vi "TPP-printer-v3.1.vi"() -> ()   [LabVIEW 2015]
uses:
  <vilib>/DAQmx/write.llb/DAQmx Write (Digital Bool 1Line 1Point).vi
  <vilib>/Utility/file.llb/Read Delimited Spreadsheet (I64).vi
  <vilib>/DAQmx/create/channels.llb/DAQmx Create Channel (DO-Digital Output).vi
  <vilib>/DAQmx/miscellaneous.llb/DAQmx Fill In Error Info.vi
  <vilib>/Platform/NI_3dgraph.lvlib
  Kinesis/Thorlabs.MotionControl.Controls.dll
panel:
  out "层时间":timestamp
  out "行时间":timestamp
  out "点时间":timestamp
  in  "f_objecitve(mm)":dbl=1.8
  in  "f_tubelens(mm)":dbl=200.0
  in  "f_scanlens(mm)":dbl=50.0
  out "%":dbl=1.1971958040155672 format="%#.2g"
  in  "读取点阵文件":path=path "C:/Users/Hongq/Desktop/grating.txt"
  in  "停止":bool
  out "每层耗时/s":dbl format="%#.2g"
  out "每行耗时/s":dbl=0.4888782501220703 format="%#.2g"
  out "每点耗时/ms":dbl=4.009246826171875 format="%#.0f"
  out "当前完成量：":u8(slide)=1 scale=0.0..100.0
  out "耗时/min":dbl=0.11883490880330404 format="%#.2g"
  out "模型XYZG坐标表":dbl[][](array[numeric])
  in  "模型高/um":dbl=1.0
  in  "总体预览":refnum<k7>(container)
  in  "刷新预览":bool
  in  "Z轴驱动序列号":string="27000001"
  in  "KCubeDCServoControl":refnum<k24>(container)
  in  "XY速度(um/s)":dbl
  out "XYZG当前值/um":dbl[](array[numeric])=[-0.4166666666666667, -0.1875, 0.0, 7.132113933563232, 7.091063499450684, 0.0] format="%#.2g"
  in  "比例因子(V/°)":dbl=0.5
  in  "AO通道：X前Y后":tag="Dev1/ao0:1"
  out "当前扫描速度(um/s)":dbl
  in  "DO通道：shutter控制":tag="Dev1/port1/line0" caption="线"
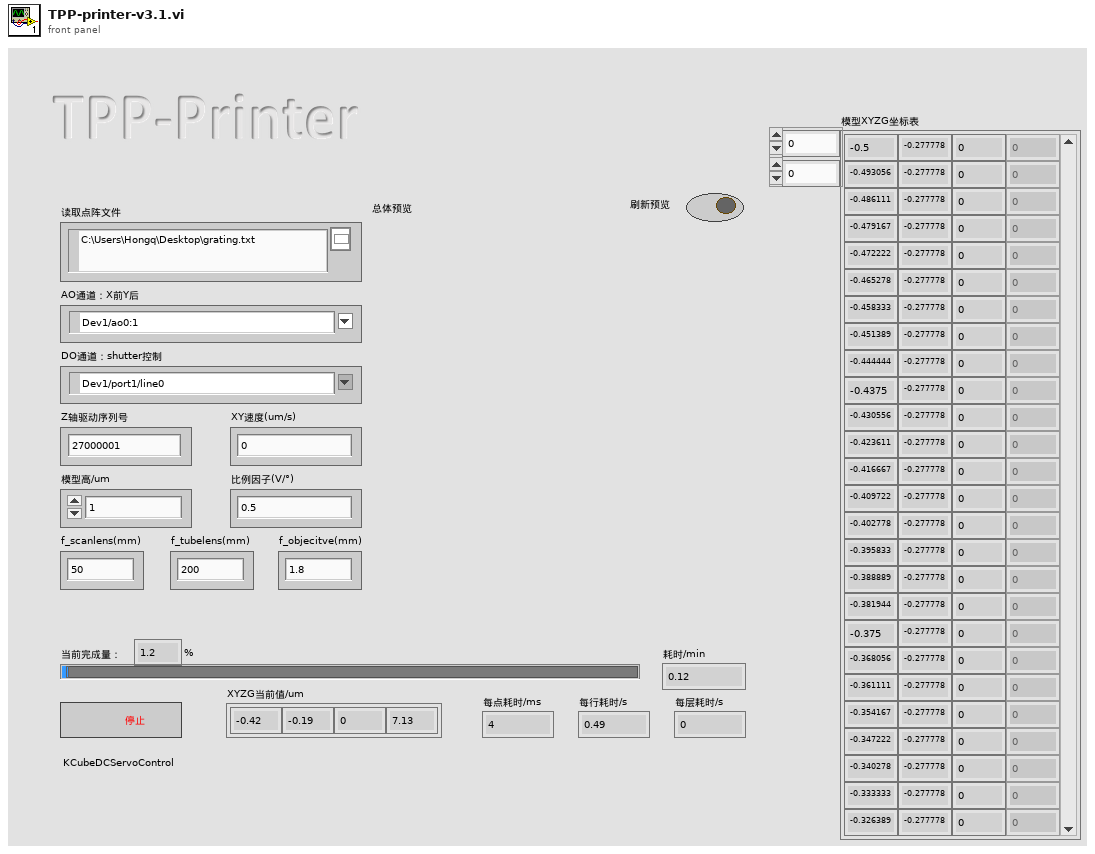
[diagram p1: front panel]
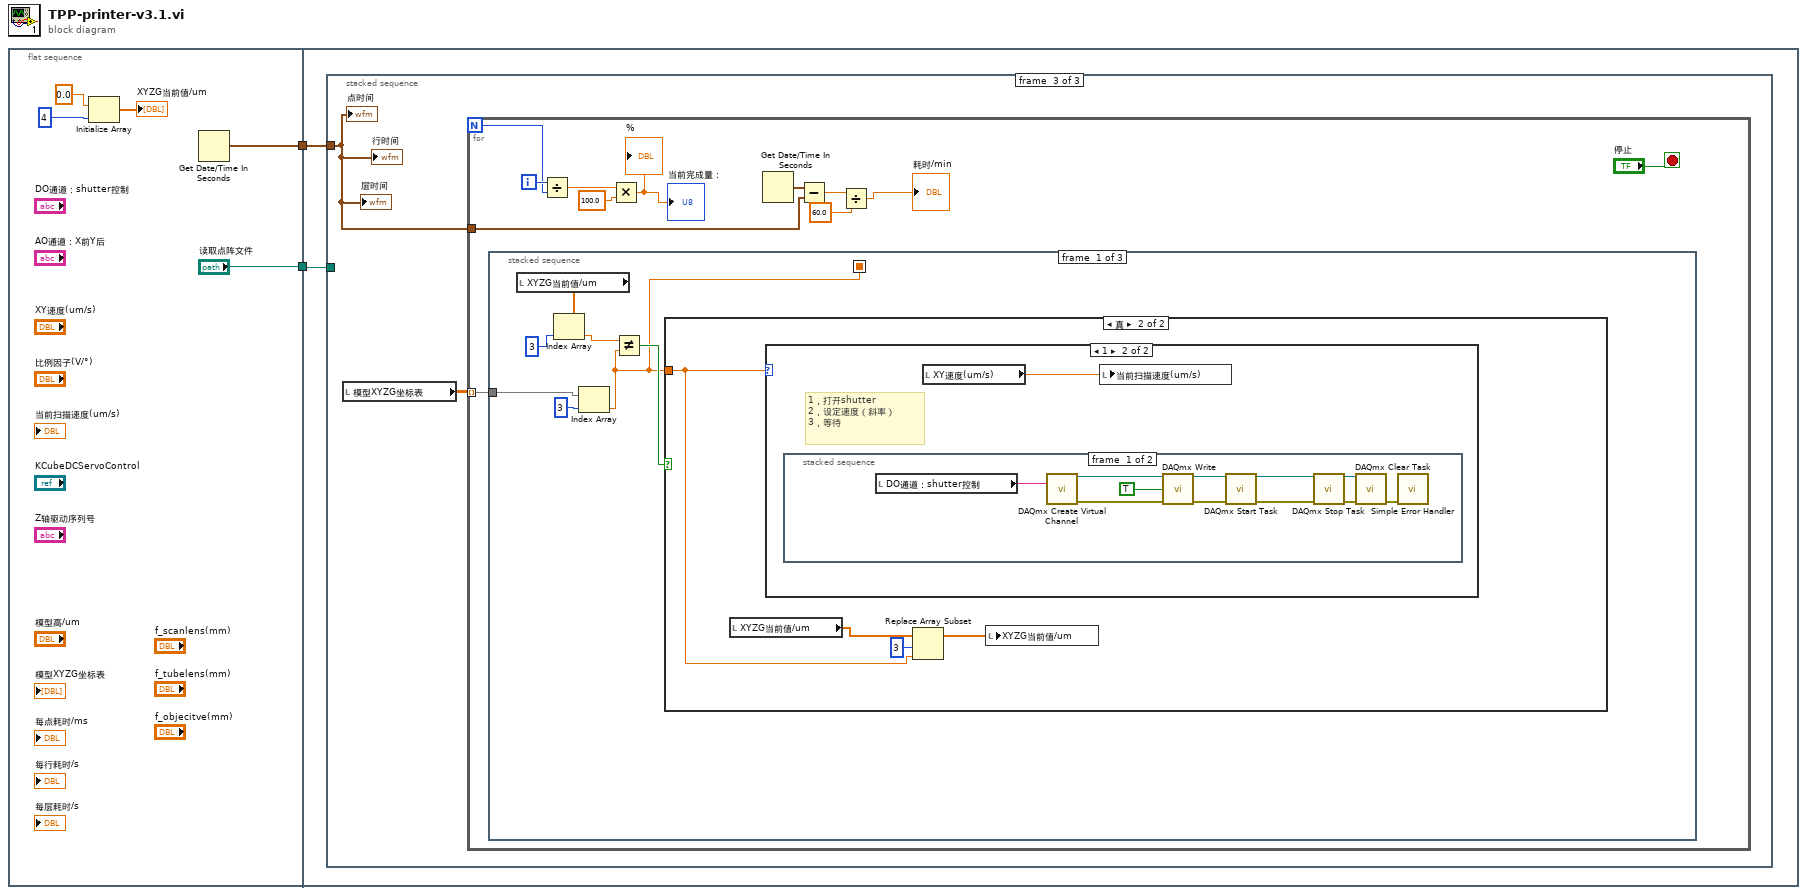
[diagram p0: block diagram]
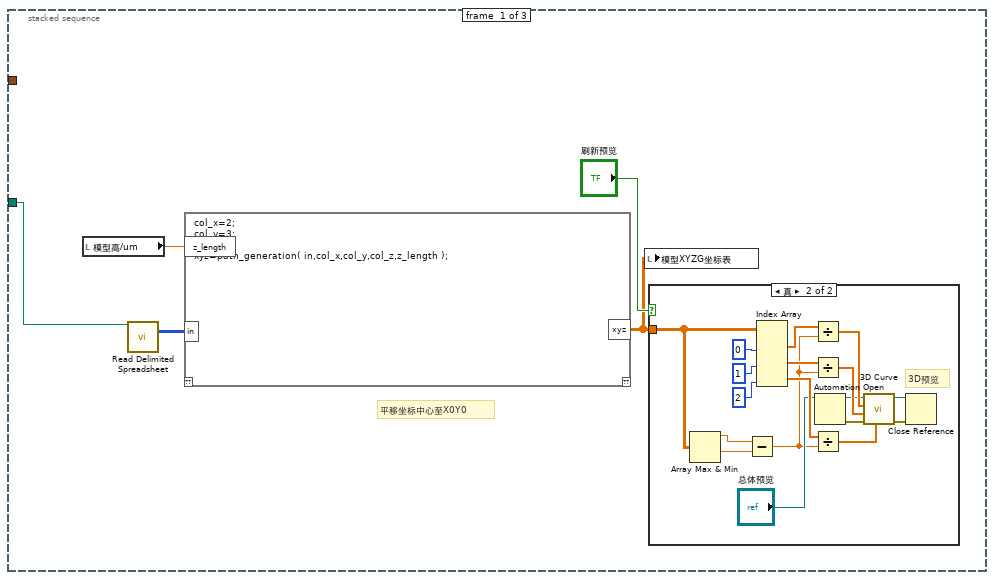
[diagram p2: hidden frame]
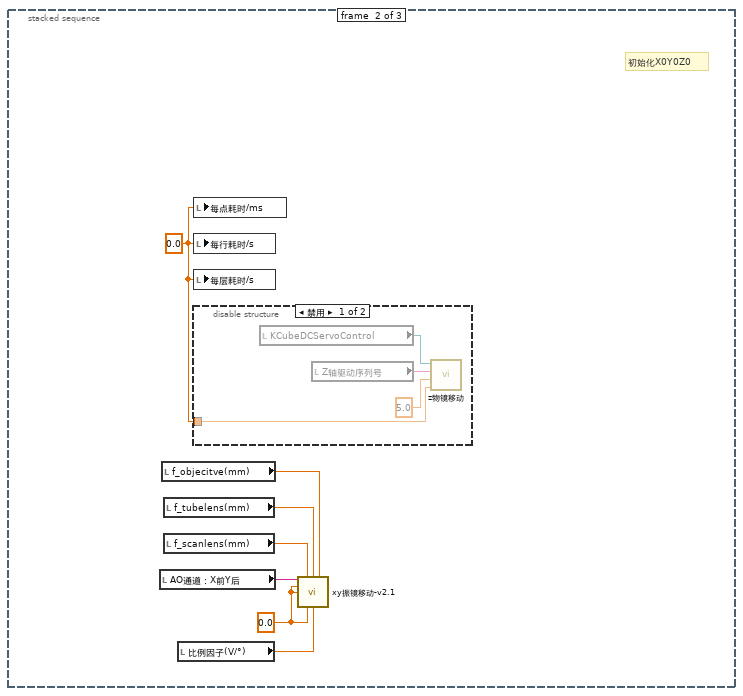
[diagram p4: hidden frame]
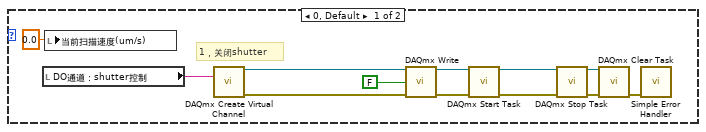
[diagram p7: hidden frame]
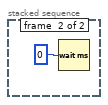
[diagram p8: hidden frame]
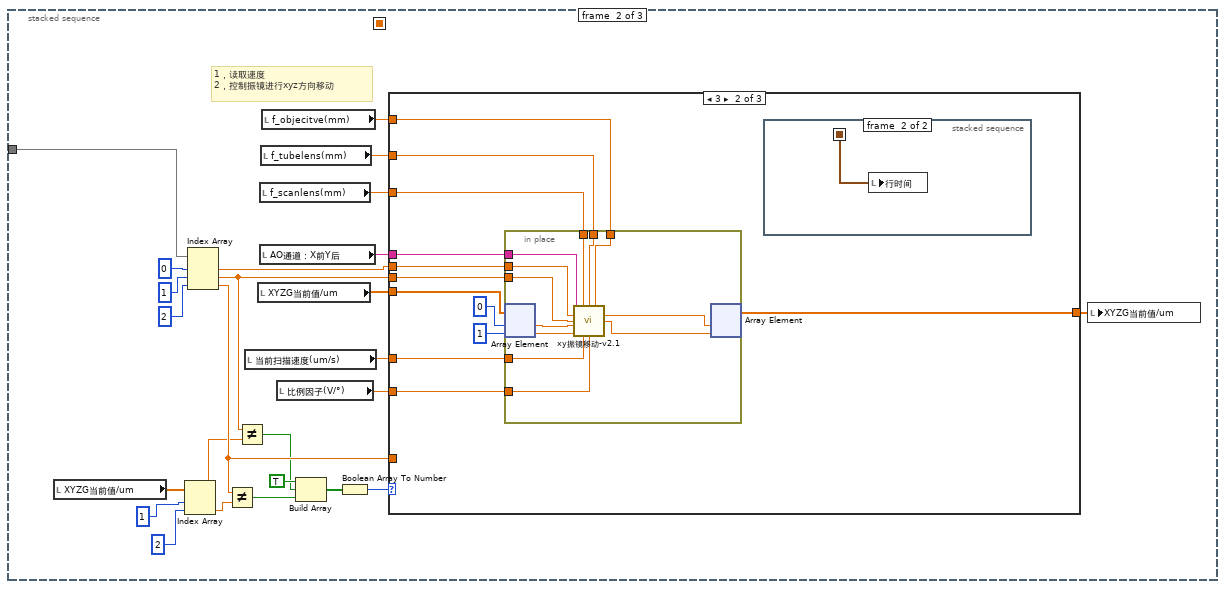
[diagram p9: hidden frame]
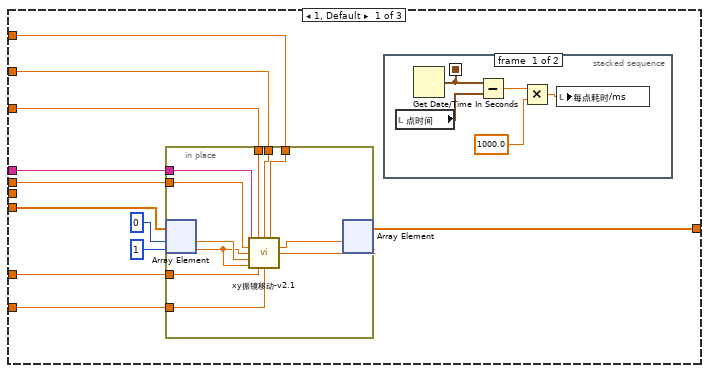
[diagram p10: hidden frame]
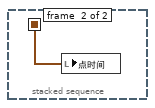
[diagram p11: hidden frame]
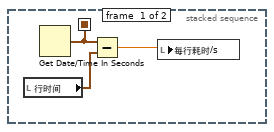
[diagram p12: hidden frame]
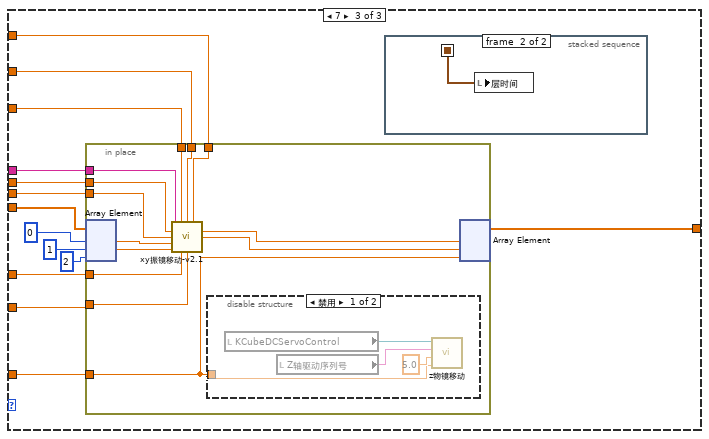
[diagram p13: hidden frame]
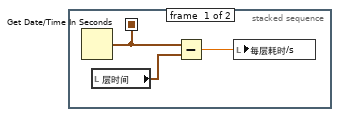
[diagram p14: hidden frame]
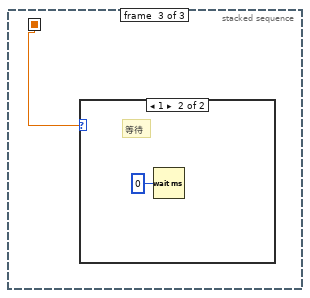
[diagram p16: hidden frame]
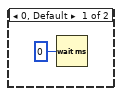
[diagram p17: hidden frame]
diagram:
  n1 = flat-sequence {
    tunnel: [w4] -> w2
    tunnel: ["读取点阵文件"] -> w1
    tunnel: w2 -> [w9]
    tunnel: w1 -> [w8]
    frame #0 {
      n2 = Initialize Array(0.0 ("元素"), 4 ("维数大小")) -> (→"XYZG当前值/um":dbl[])
      n3 = Get Date/Time In Seconds() -> (seconds since 1Jan1904=w4:timestamp)
    }
    frame #1 {
      n4 = stacked-sequence {
        tunnel: w9 -> [_ _ w44]
        tunnel: w8 -> [w13 _ _]
        frame #0 {
          # "平移坐标中心至X0Y0"
          n5 = local read "模型高/um"() -> (w11:dbl)
          n6 = call-poly <vilib>:"Read Delimited Spreadsheet.vi"("file path (dialog if empty)"=w13) -> ("all rows"=w12:i64[][])  [unwired: 9 in, 5 out]
          n7 = script code="col_x=2;\ncol_y=3;\ncol_z=4;\nxyz=path_generation( in,col_x,col_y,col_z,z_length );"("in"=w12, "z_length"=w11) -> ("xyz"=w10:dbl[][])  [unwired: 1 in, 1 out]
          n8 = local write "模型XYZG坐标表"(w10) -> ()
          n9 = case shown="真" "刷新预览" {
            tunnel: w10 -> [_ w18]
            frame False {
            }
            frame True {
              # "3D预览"
              n10 = Array Max & Min(array=w18) -> (max value=w16:dbl, min value=w17:dbl)  [unwired: 2 out]
              n11 = Subtract(x=w16, y=w17) -> (x-y=w15:dbl)
              n12 = Index Array(array=w18, index (col) #1=0 ("禁用的索引 (列)"), index (col) #2=1 ("索引 (列)"), index (col) #3=2 ("索引 (列)")) -> (element #1=w29:dbl[], element #2=w28:dbl[], element #3=w27:dbl[])  [unwired: 3 in]
              n13 = Divide(x=w29, y=w15) -> (x/y=w24:dbl[])
              n14 = Divide(x=w28, y=w15) -> (x/y=w25:dbl[])
              n15 = Divide(x=w27, y=w15) -> (x/y=w26:dbl[])
              n16 = Automation Open(Automation Refnum="总体预览") -> (Automation Refnum=w22:refnum<k7>, error out=w19:errorcluster)  [unwired: 3 in]
              n17 = call <vilib>:"3D Curve.vi"("z vector"=w26, "error in (no error)"=w19, "y vector"=w25, "x vector"=w24, "3D graph"=w22) -> ("error out"=w21:errorcluster, "3D graph out"=w20:refnum<k7>)  [unwired: 5 in]
              n18 = Close Reference(reference=w20, error in (no error)=w21) -> ()  [unwired: 1 out]
            }
          }
        }
        frame #1 {
          w34 = 0.0 ("每点耗时/ms")
          w33 = 0.0 ("速度(°/s)")
          # "初始化X0Y0Z0"
          n19 = local read "AO通道：X前Y后"() -> (w39:tag)
          n20 = local read "f_objecitve(mm)"() -> (w35:dbl)
          n21 = local read "f_tubelens(mm)"() -> (w36:dbl)
          n22 = local read "f_scanlens(mm)"() -> (w37:dbl)
          n23 = local read "比例因子(V/°)"() -> (w38:dbl)
          n24 = local write "每点耗时/ms"(w34) -> ()
          n25 = local write "每行耗时/s"(w34) -> ()
          n26 = local write "每层耗时/s"(w34) -> ()
          n27 = disable-structure shown="禁用" {
            disable-tunnel: w34 -> [w40 _]
            frame Disabled {
              n28 = local read "KCubeDCServoControl"() -> (w43:refnum<k24>)
              n29 = local read "Z轴驱动序列号"() -> (w42:string)
              n30 = call "z物镜移动.vi"("position"=w40, "maxVelocity"=5.0, "SerialNumber"=w42, "KCubeDCServoControl"=w43) -> ()  [unwired: 5 in, 3 out]
            }
            frame Enabled {
            }
          }
          n31 = call "xy振镜移动-v2.1.vi"("AO通道：X前Y后"=w39, "f_scanlens(mm)"=w37, "f_tubelens(mm)"=w36, "f_objecitve(mm)"=w35, "x终止位(um)"=w33, "y终止位(um)"=w33, "速度(um/s)"=w33, "比例因子(V/°)"=w38) -> ()  [unwired: 6 in, 2 out]
        }
        frame #2 {
          n32 = local read "模型XYZG坐标表"() -> (w45:dbl[][])
          n33 = for {
            N -> [w55]
            tunnel: w45 -> [w57] mode=indexing
            tunnel: w44 -> [w51]
            i -> [w56]
            stop <- "停止" stop-if-true
            n34 = stacked-sequence {
              seq-local: [w58 _ _] -> [_ _ w210]
              tunnel: w57 -> [w63 w117 _]
              frame #0 {
                n35 = local read "XYZG当前值/um"() -> (w61:dbl[])
                n36 = Index Array(array=w61, index=3 ("索引")) -> (element=w59:dbl)
                n37 = Index Array(array=w63, index=3 ("禁用的索引 (列)")) -> (element=w58:dbl)
                n38 = Not Equal?(x=w59, y=w58) -> (x != y?=w62:bool)
                n39 = case shown="真" w62 {
                  tunnel: w58 -> [_ w66]
                  frame False {
                  }
                  frame True {
                    n40 = local read "XYZG当前值/um"() -> (w68:dbl[])
                    n41 = case shown="1" w66 {
                      frame 0, Default {
                        # "1，关闭shutter"
                        n42 = local read "DO通道：shutter控制"() -> (w72:tag)
                        n43 = local write "当前扫描速度(um/s)"(0.0 ("扫描速度(°/s)")) -> ()
                        n44 = call-poly <vilib>:"DAQmx Create Virtual Channel.vi"("lines"=w72) -> ("task out"=w80:refnum<k21>, "error out"=w79:errorcluster)  [unwired: 13 in]
                        n45 = call-poly <vilib>:"DAQmx Write.vi"("task/channels in"=w80, "data"=FALSE, "error in"=w79) -> ("task out"=w77:refnum<k21>, "error out"=w76:errorcluster)  [unwired: 10 in, 1 out]
                        n46 = call <vilib>:"DAQmx Start Task.vi"("task/channels in"=w77, "error in"=w76) -> ("task out"=w70:refnum<k21>, "error out"=w69:errorcluster)  [unwired: 12 in]
                        n47 = call <vilib>:"DAQmx Stop Task.vi"("task/channels in"=w70, "error in"=w69) -> ("task out"=w75:refnum<k21>, "error out"=w74:errorcluster)  [unwired: 12 in]
                        n48 = call <vilib>:"DAQmx Clear Task.vi"("task in"=w75, "error in"=w74) -> ("error out"=w73:errorcluster)  [unwired: 13 in]
                        n49 = call <vilib>:"Simple Error Handler.vi"("error in (no error)"=w73) -> ()  [unwired: 4 in, 5 out]
                      }
                      frame 1 {
                        # "1，打开shutter\n2，设定速度（斜率）\n3，等待"
                        n50 = stacked-sequence {
                          frame #0 {
                            n51 = local read "DO通道：shutter控制"() -> (w84:tag)
                            n52 = call-poly <vilib>:"DAQmx Create Virtual Channel.vi"("lines"=w84) -> ("task out"=w92:refnum<k21>, "error out"=w91:errorcluster)  [unwired: 13 in]
                            n53 = call-poly <vilib>:"DAQmx Write.vi"("task/channels in"=w92, "data"=TRUE, "error in"=w91) -> ("task out"=w89:refnum<k21>, "error out"=w88:errorcluster)  [unwired: 10 in, 1 out]
                            n54 = call <vilib>:"DAQmx Start Task.vi"("task/channels in"=w89, "error in"=w88) -> ("task out"=w83:refnum<k21>, "error out"=w82:errorcluster)  [unwired: 12 in]
                            n55 = call <vilib>:"DAQmx Stop Task.vi"("task/channels in"=w83, "error in"=w82) -> ("task out"=w87:refnum<k21>, "error out"=w86:errorcluster)  [unwired: 12 in]
                            n56 = call <vilib>:"DAQmx Clear Task.vi"("task in"=w87, "error in"=w86) -> ("error out"=w85:errorcluster)  [unwired: 13 in]
                            n57 = call <vilib>:"Simple Error Handler.vi"("error in (no error)"=w85) -> ()  [unwired: 4 in, 5 out]
                          }
                          frame #1 {
                            n58 = Wait (ms)(milliseconds to wait=u32 0 ("等待时间（毫秒）")) -> ()  [unwired: 1 out]
                          }
                        }
                        n59 = local read "XY速度(um/s)"() -> (w81:dbl)
                        n60 = local write "当前扫描速度(um/s)"(w81) -> ()
                      }
                    }
                    n61 = Replace Array Subset(array=w68, new element=w66, index=3 ("索引")) -> (w65:dbl[])
                    n62 = local write "XYZG当前值/um"(w65) -> ()
                  }
                }
              }
              frame #1 {
                # "1，读取速度\n2，控制振镜进行xyz方向移动"
                n63 = local read "XYZG当前值/um"() -> (w104:dbl[])
                n64 = Index Array(array=w104, index #1=1 ("索引"), index #2=2 ("索引")) -> (element #1=w95:dbl, element #2=w97:dbl)
                n65 = Index Array(array=w117, index #1=0 ("禁用的索引 (列)"), index #2=1 ("索引"), index #3=2 ("索引")) -> (element #1=w108:dbl, element #2=w96:dbl, element #3=w103:dbl)
                n66 = Not Equal?(x=w103, y=w97) -> (x != y?=w102:bool)
                n67 = Not Equal?(x=w96, y=w95) -> (x != y?=w94:bool)
                n68 = local read "当前扫描速度(um/s)"() -> (w114:dbl)
                n69 = local read "XYZG当前值/um"() -> (w112:dbl[])
                n70 = local read "f_scanlens(mm)"() -> (w101:dbl)
                n71 = local read "AO通道：X前Y后"() -> (w116:tag)
                n72 = local read "f_tubelens(mm)"() -> (w100:dbl)
                n73 = local read "f_objecitve(mm)"() -> (w99:dbl)
                n74 = local read "比例因子(V/°)"() -> (w115:dbl)
                n75 = Build Array(TRUE ("元素"), w94, w102) -> (w110:bool[])
                n76 = Boolean Array To Number(Boolean array=w110) -> (number=w111:u32)
                n77 = case shown="3" w111 {
                  tunnel: w116 -> [w124 w153 w185]
                  tunnel: w115 -> [w123 w152 w186]
                  tunnel: w108 -> [w126 w154 w184]
                  tunnel: w112 -> [w129 w155 w183]
                  tunnel: [w119 w147 w175] -> w113
                  tunnel: w114 -> [w125 w156 w182]
                  tunnel: w96 -> [_ w151 w181]
                  tunnel: w103 -> [_ _ w176]
                  tunnel: w101 -> [w122 w150 w180]
                  tunnel: w100 -> [w121 w149 w179]
                  tunnel: w99 -> [w120 w148 w178]
                  frame 1, Default {
                    n78 = in-place {
                      in-place-border: w126 -> [w140]
                      in-place-border: w125 -> [w146]
                      in-place-border: w124 -> [w145]
                      in-place-border: w123 -> [w144]
                      in-place-border: w122 -> [w143]
                      in-place-border: w121 -> [w142]
                      in-place-border: w120 -> [w141]
                      n79 = in-place-array #1(w129, 0, 1) -> (w139:dbl, w138:dbl)
                      n80 = call "xy振镜移动-v2.1.vi"("AO通道：X前Y后"=w145, "f_scanlens(mm)"=w143, "f_tubelens(mm)"=w142, "f_objecitve(mm)"=w141, "x终止位(um)"=w140, "y终止位(um)"=w138, "x初始位(um)"=w139, "y初始位(um)"=w138, "速度(um/s)"=w146, "比例因子(V/°)"=w144) -> ("x终止位(um) 2"=w137:dbl, "y终止位(um) 2"=w136:dbl)  [unwired: 4 in]
                      n81 = in-place-array #1(w137, w136) -> (w119:dbl[])  [unwired: 2 out]
                    }
                    n82 = stacked-sequence {
                      seq-local: [w130 _] -> [_ w135]
                      frame #0 {
                        n83 = local read "点时间"() -> (w131:timestamp)
                        n84 = Get Date/Time In Seconds() -> (seconds since 1Jan1904=w130:timestamp)
                        n85 = Subtract(x=w130, y=w131) -> (x-y=w134:dbl)
                        n86 = Multiply(x=w134, y=1000.0) -> (x*y=w132:dbl)
                        n87 = local write "每点耗时/ms"(w132) -> ()
                      }
                      frame #1 {
                        n88 = local write "点时间"(w135) -> ()
                      }
                    }
                  }
                  frame 3 {
                    n89 = in-place {
                      in-place-border: w154 -> [w174]
                      in-place-border: w156 -> [w173]
                      in-place-border: w153 -> [w172]
                      in-place-border: w152 -> [w171]
                      in-place-border: w151 -> [w167]
                      in-place-border: w150 -> [w170]
                      in-place-border: w149 -> [w169]
                      in-place-border: w148 -> [w168]
                      n90 = in-place-array #2(w155, 0, 1) -> (w166:dbl, w165:dbl)
                      n91 = call "xy振镜移动-v2.1.vi"("AO通道：X前Y后"=w172, "f_scanlens(mm)"=w170, "f_tubelens(mm)"=w169, "f_objecitve(mm)"=w168, "x终止位(um)"=w174, "y终止位(um)"=w167, "x初始位(um)"=w166, "y初始位(um)"=w165, "速度(um/s)"=w173, "比例因子(V/°)"=w171) -> ("x终止位(um) 2"=w164:dbl, "y终止位(um) 2"=w163:dbl)  [unwired: 4 in]
                      n92 = in-place-array #2(w164, w163) -> (w147:dbl[])  [unwired: 2 out]
                    }
                    n93 = stacked-sequence {
                      seq-local: [w159 _] -> [_ w162]
                      frame #0 {
                        n94 = local read "行时间"() -> (w161:timestamp)
                        n95 = Get Date/Time In Seconds() -> (seconds since 1Jan1904=w159:timestamp)
                        n96 = Subtract(x=w159, y=w161) -> (x-y=w160:dbl)
                        n97 = local write "每行耗时/s"(w160) -> ()
                      }
                      frame #1 {
                        n98 = local write "行时间"(w162) -> ()
                      }
                    }
                  }
                  frame 7 {
                    n99 = in-place {
                      in-place-border: w184 -> [w204]
                      in-place-border: w182 -> [w195]
                      in-place-border: w185 -> [w205]
                      in-place-border: w186 -> [w194]
                      in-place-border: w181 -> [w203]
                      in-place-border: w180 -> [w198]
                      in-place-border: w179 -> [w197]
                      in-place-border: w178 -> [w196]
                      in-place-border: w176 -> [w193]
                      n100 = in-place-array #3(w183, 0, 1, 2) -> (w200:dbl, w199:dbl)  [unwired: 1 out]
                      n101 = call "xy振镜移动-v2.1.vi"("AO通道：X前Y后"=w205, "f_scanlens(mm)"=w198, "f_tubelens(mm)"=w197, "f_objecitve(mm)"=w196, "x终止位(um)"=w204, "y终止位(um)"=w203, "x初始位(um)"=w200, "y初始位(um)"=w199, "速度(um/s)"=w195, "比例因子(V/°)"=w194) -> ("x终止位(um) 2"=w202:dbl, "y终止位(um) 2"=w201:dbl)  [unwired: 4 in]
                      n102 = disable-structure shown="禁用" {
                        disable-tunnel: w193 -> [w206 _]
                        frame Disabled {
                          n103 = local read "KCubeDCServoControl"() -> (w209:refnum<k24>)
                          n104 = local read "Z轴驱动序列号"() -> (w208:string)
                          n105 = call "z物镜移动.vi"("position"=w206, "maxVelocity"=5.0, "SerialNumber"=w208, "KCubeDCServoControl"=w209) -> ()  [unwired: 5 in, 3 out]
                        }
                        frame Enabled {
                        }
                      }
                      n106 = in-place-array #3(w202, w201, w193) -> (w175:dbl[])  [unwired: 3 out]
                    }
                    n107 = stacked-sequence {
                      seq-local: [w190 _] -> [_ w192]
                      frame #0 {
                        n108 = Get Date/Time In Seconds() -> (seconds since 1Jan1904=w190:timestamp)
                        n109 = local read "层时间"() -> (w189:timestamp)
                        n110 = Subtract(x=w190, y=w189) -> (x-y=w191:dbl)
                        n111 = local write "每层耗时/s"(w191) -> ()
                      }
                      frame #1 {
                        n112 = local write "层时间"(w192) -> ()
                      }
                    }
                  }
                }
                n113 = local write "XYZG当前值/um"(w113) -> ()
              }
              frame #2 {
                n114 = case shown="1" w210 {
                  frame 0, Default {
                    n115 = Wait (ms)(milliseconds to wait=u32 0 ("等待时间（毫秒）")) -> ()  [unwired: 1 out]
                  }
                  frame 1 {
                    # "等待"
                    n116 = Wait (ms)(milliseconds to wait=u32 0 ("等待时间（毫秒）")) -> ()  [unwired: 1 out]
                  }
                }
              }
            }
            n117 = Divide(x=w56, y=w55) -> (x/y=w54:dbl)
            n118 = Multiply(x=w54, y=100.0) -> (x*y=→"当前完成量：" →"%":dbl)
            n119 = Get Date/Time In Seconds() -> (seconds since 1Jan1904=w46:timestamp)
            n120 = Subtract(x=w46, y=w51) -> (x-y=w49:dbl)
            n121 = Divide(x=w49, y=60.0) -> (x/y=→"耗时/min":dbl)
          }
          "点时间" <- w44
          "行时间" <- w44
          "层时间" <- w44
        }
      }
    }
  }
